vi "Rename Digital Pattern From FPGA Resource.vi"(6 "Old FPGA Resource":string, 8 "error in (no error)":errorcluster, 9 "New FPGA Resource":string, 10 "Page Data in":T1 {"Node Ptr" format="%.0x"}, 11 "State Queue in":string[](array[string])) -> (0 "error out":errorcluster, 2 "Page Data out":T1 {"Node Ptr" format="%.0x"}, 3 "State Queue out":string[](array[string]))   [LabVIEW 2017, in "Engine Simulation Toolkit System Explorer.lvlib"]
uses:
  Engine Simulation Toolkit System Explorer.lvlib
  Digital Patterns Page Data.ctl
  <vilib>/NI Veristand/Custom Device API/Custom Device Item Ref.ctl
  Digital Pattern.ctl
  Digital Pattern Base.ctl
  Digital Pattern Remove Edge.ctl
  Digital Pattern Add Pulse.ctl
  <vilib>/NI Veristand/Custom Device API/Custom Device API.lvlib
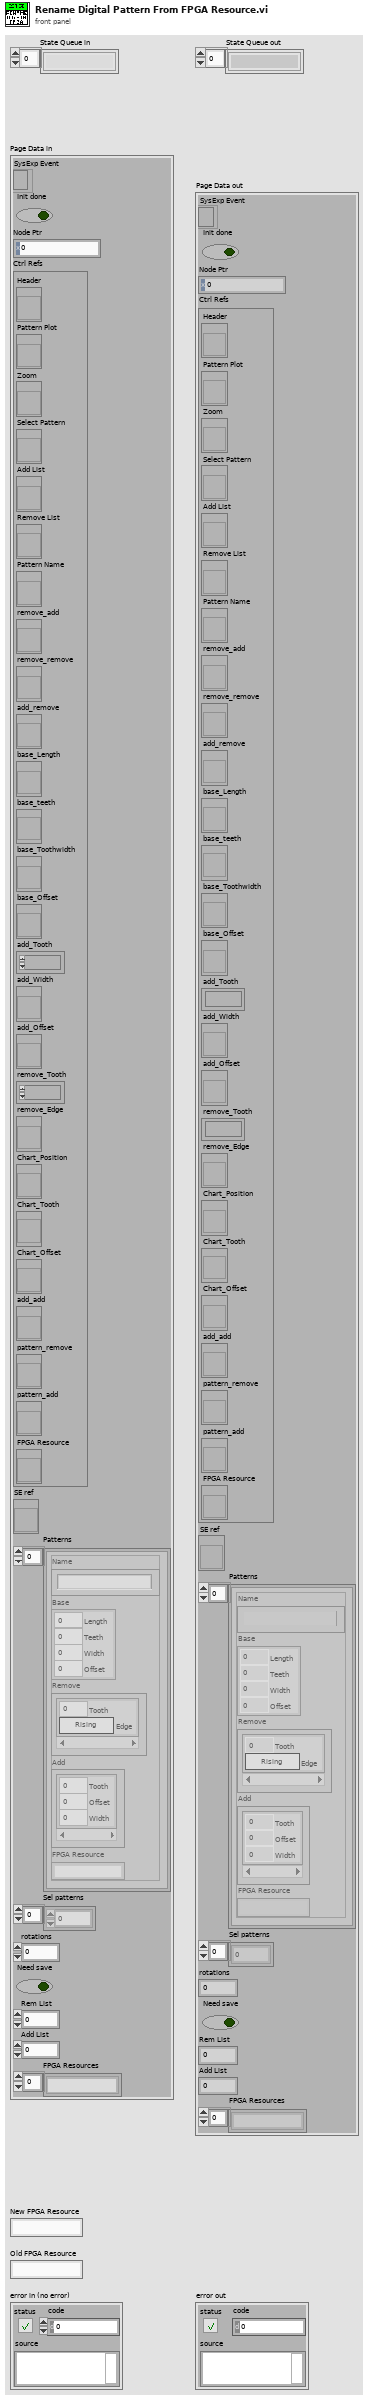
[diagram p1: front panel]
types:
  T1 = typedef "Engine Simulation Toolkit System Explorer.lvlib/Digital Patterns Page Data.ctl" = cluster{"SysExp Event":refnum<event-registration>, "Init done":bool, "Node Ptr":T2, "Ctrl Refs":cluster{"Header":refnum<vi>, "Pattern Plot":refnum<vi>, "Zoom":refnum<vi>, "Select Pattern":refnum<vi>, "Add List":refnum<vi>, "Remove List":refnum<vi>, "Pattern Name":refnum<vi>, "remove_add":refnum<vi>, "remove_remove":refnum<vi>, "add_remove":refnum<vi>, "base_Length":refnum<vi>, "base_teeth":refnum<vi>, "base_Toothwidth":refnum<vi>, "base_Offset":refnum<vi>, "add_Tooth":refnum<vi>, "add_Width":refnum<vi>, "add_Offset":refnum<vi>, "remove_Tooth":refnum<vi>, "remove_Edge":refnum<vi>, "Chart_Position":refnum<vi>, "Chart_Tooth":refnum<vi>, "Chart_Offset":refnum<vi>, "add_add":refnum<vi>, "pattern_remove":refnum<vi>, "pattern_add":refnum<vi>, "FPGA Resource":refnum<vi>}, "SE ref":refnum<vi>, "Patterns":T3[], "Sel patterns":i32[], "rotations":u16, "Need save":bool, "Rem List":i32, "Add List":i32, "FPGA Resources":string[]}
  T2 = typedef "Custom Device API.lvlib/Custom Device Item Ref.ctl" = u64
  T3 = typedef "Engine Simulation Toolkit System Explorer.lvlib/Digital Pattern.ctl" = cluster{"Name":string, "Base":T4, "Remove":T5[], "Add":T6[], "FPGA Resource":string}
  T4 = typedef "Engine Simulation Toolkit System Explorer.lvlib/Digital Pattern Base.ctl" = cluster{"Length":dbl, "Teeth":u16, "Width":dbl, "Offset":dbl}
  T5 = typedef "Engine Simulation Toolkit System Explorer.lvlib/Digital Pattern Remove Edge.ctl" = cluster{"Tooth":u16, "Edge":bool}
  T6 = typedef "Engine Simulation Toolkit System Explorer.lvlib/Digital Pattern Add Pulse.ctl" = cluster{"Tooth":u16, "Offset":dbl, "Width":dbl}
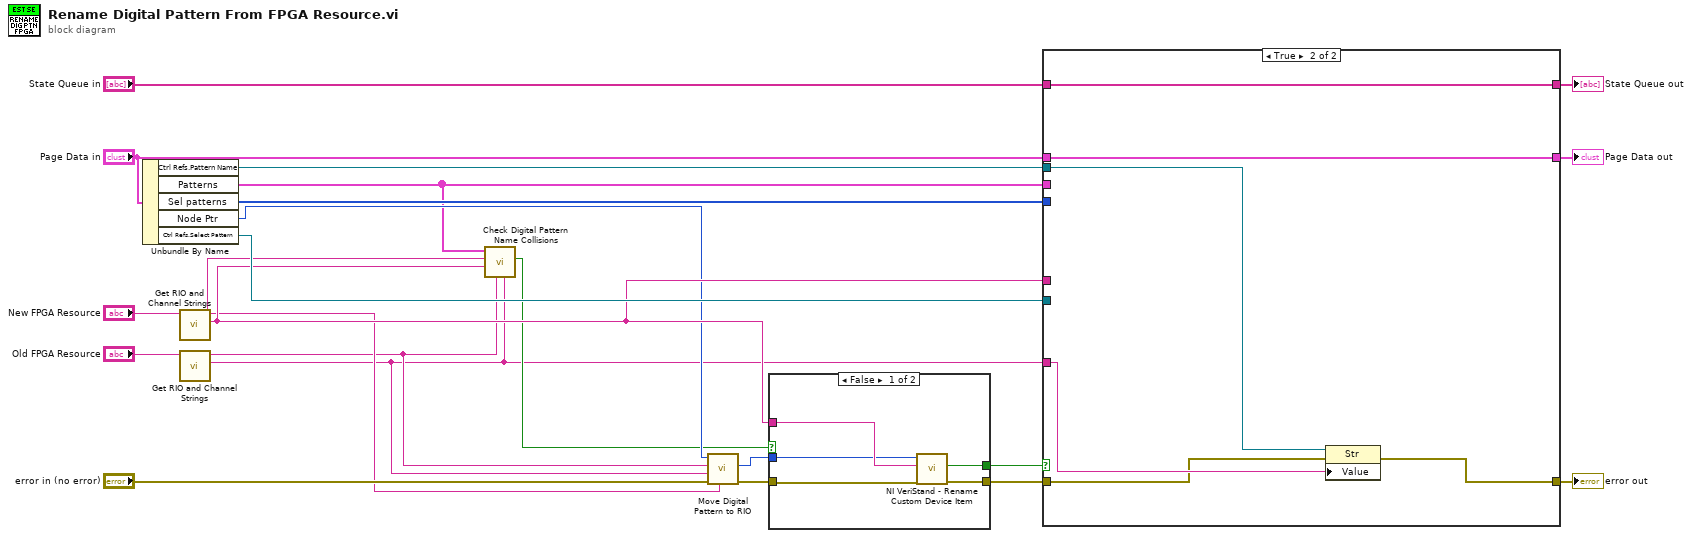
[diagram p0: block diagram]
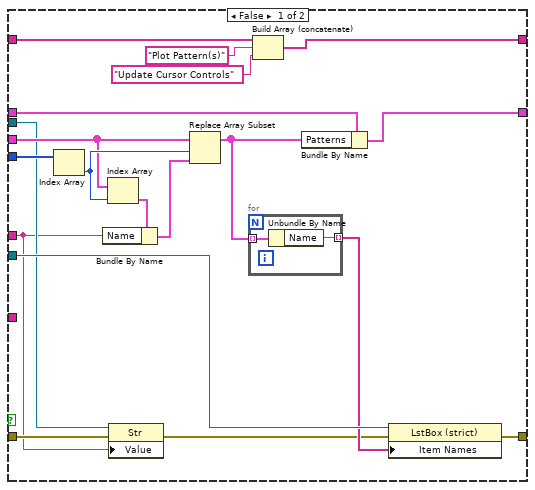
[diagram p3: hidden frame]
diagram:
  n1 = Unbundle By Name("Page Data in") -> ("Ctrl Refs.Pattern Name"=w16:refnum<vi>, "Patterns"=w3:T3[], "Sel patterns"=w18:i32[], "Node Ptr"=w7:T2, "Ctrl Refs.Select Pattern"=w13:refnum<vi>)
  n2 = call "Get RIO and Channel Strings.vi"("rio/channel"="New FPGA Resource") -> ("channel"=w11:string, "rio"=w5:string)  [unwired: 9 in]
  n3 = call "Get RIO and Channel Strings.vi"("rio/channel"="Old FPGA Resource") -> ("channel"=w1:string, "rio"=w2:string)  [unwired: 9 in]
  n4 = call "Check Digital Pattern Name Collisions.vi"("old name"=w1, "old rio"=w2, "new name"=w11, "new rio"=w5, "Patterns"=w3) -> ("name collision?"=w4:bool)  [unwired: 5 in, 1 out]
  n5 = call "Move Digital Pattern to RIO.vi"("New RIO"=w5, "error in (no error)"="error in (no error)", "Name"=w1, "Old RIO"=w2, "Item Ref in"=w7) -> ("error out"=w8:errorcluster, "Digital Pattern Ref out"=w6:T2)  [unwired: 4 in, 1 out]
  n6 = case shown="False" w4 {
    selector: w4 -> [_ w28]
    tunnel: w8 -> [w24 w29]
    tunnel: w6 -> [w23 _]
    tunnel: [w27 w29] -> w15
    tunnel: w11 -> [w25 _]
    tunnel: [w26 w28] -> w14
    frame False {
      n7 = call <vilib>:"NI VeriStand - Rename Custom Device Item.vi"("error in (no error)"=w24, "New Name"=w25, "Item Ref in"=w23) -> ("error out"=w27:errorcluster, "Request invalid?"=w26:bool)  [unwired: 6 in, 1 out]
    }
    frame True {
    }
  }
  n8 = case shown="True" w14 {
    tunnel: "State Queue in" -> [w48 w55]
    tunnel: w3 -> [w44 _]
    tunnel: w18 -> [w43 _]
    tunnel: "Page Data in" -> [w42 w54]
    tunnel: [w41 w54] -> w20
    tunnel: [w40 w55] -> w21
    tunnel: w1 -> [_ w56]
    tunnel: w11 -> [w30 _]
    tunnel: [w36 w51] -> w22
    tunnel: w15 -> [w33 w52]
    tunnel: w16 -> [w31 w53]
    tunnel: w13 -> [w35 _]
    frame False {
      n9 = Index Array(array=w43) -> (element=w45:i32)  [unwired: 1 in]
      n10 = Index Array(array=w44, index=w45) -> (element=w46:T3)
      n11 = Bundle By Name(cluster=w46, "Name"=w30) -> (w47:T3)
      n12 = property class="Str"(reference=w31, error in=w33, "Value"=w30) -> (error out=w32:errorcluster)  [unwired: 1 out]
      n13 = Replace Array Subset(array=w44, new element=w47, index=w45) -> (w37:T3[])
      n14 = for {
        tunnel: w37 -> [w50] mode=indexing
        tunnel: [w49] -> w34 mode=indexing
        n15 = Unbundle By Name(w50) -> ("Name"=w49:string)
      }
      n16 = Build Array (concatenate)(w48, "Plot Pattern(s)", "Update Cursor Controls") -> (w40:string[])
      n17 = Bundle By Name(cluster=w42, "Patterns"=w37) -> (w41:T1)
      n18 = property class="LstBox (strict)"(reference=w35, error in=w32, "Item Names"=w34) -> (error out=w36:errorcluster)  [unwired: 1 out]
    }
    frame True {
      n19 = property class="Str"(reference=w53, error in=w52, "Value"=w56) -> (error out=w51:errorcluster)  [unwired: 1 out]
    }
  }
  "error out" <- w22
  "State Queue out" <- w21
  "Page Data out" <- w20
